vi "Edit User FIR.vi"(0 "VISA Resource Name":refnum<visa-resource-name>, 5 "File Name (FIR_DATA)":string="FIR_DATA", 7 "Coefficient Value":dbl[](array[numeric]) format="%.2f", 9 "Oversample Ratio (4)":i32=4, 11 "error in (no error)":errorcluster {"code" format="%.0x"}) -> (4 "VISA Resource Name Out":refnum<visa-resource-name>, 15 "error out":errorcluster {"code" format="%.0x"})   [LabVIEW 2012, in "Agilent ESG Series.lvlib"]
doc: "This VI is used to define user FIR filters. A maximun filter length of 1024 taps is allowed with a maximum oversampling ratio of 32.\nA FIR selected for use in CDMA cannot have more than 256 taps.\n\nThis VI is valid only on instruments E44xxB with the UND and UN5 options or option 101 or on instrument E4438C with option 001/601 or 002/602."
uses:
  <instrlib>/Agilent ESG Series/Agilent ESG Series.lvlib
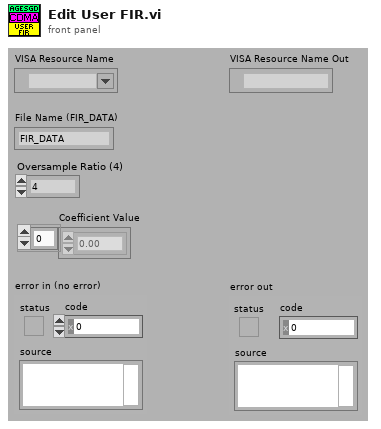
[diagram p1: front panel]
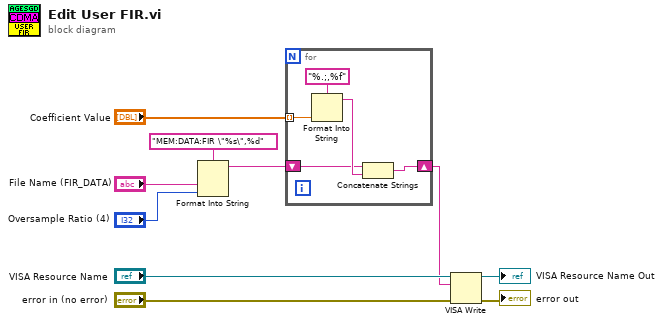
[diagram p0: block diagram]
diagram:
  n1 = Format Into String(format string="MEM:DATA:FIR \"%s\",%d" ("string (\"\")"), "File Name (FIR_DATA)", "Oversample Ratio (4)") -> (resulting string=w4:string)  [unwired: 2 in, 1 out]
  n2 = for {
    tunnel: "Coefficient Value" -> [w14] mode=indexing
    shift-right: [w13] -> w3
    shift-left: w4 -> [w12]
    n3 = Format Into String(format string="%.;,%f", w14) -> (resulting string=w15:string)  [unwired: 2 in, 1 out]
    n4 = Concatenate Strings(w12, w15) -> (w13:string)
  }
  n5 = VISA Write(VISA resource name="VISA Resource Name", write buffer=w3, error in (no error)="error in (no error)") -> (VISA resource name out=→"VISA Resource Name Out":refnum<visa-resource-name>, error out=→"error out":errorcluster)  [unwired: 1 out]
